vi "3_3_(2).vi"() -> ()   [LabVIEW 2012]
uses:
  Control 1.ctl
panel:
  in  "Таблиця 1 - Вхідні дані":string[][](table)
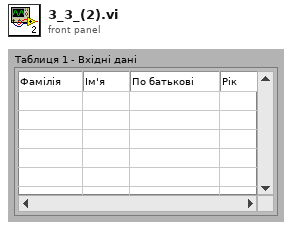
[diagram p1: front panel]
types:
  T1 = typedef "Control 1.ctl" = enum16{"Серверу", "Клієнту", "Зчитати", "Стоп", "1", "2", "3", "4"}
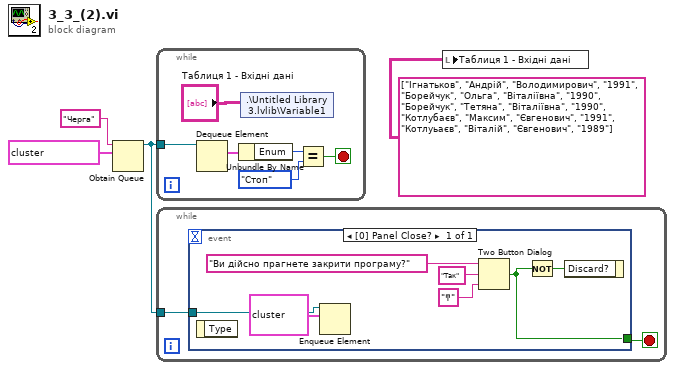
[diagram p0: block diagram]
diagram:
  n1 = Obtain Queue(name (unnamed)="Черга", element data type=cluster{"variant":variant, "Enum":T1} {"variant"=variant, "Enum"=enum."Стоп"}) -> (queue out=w2:refnum<queue>)  [unwired: 3 in, 2 out]
  n2 = while {
    tunnel: w2 -> [w10]
    stop <- w7 stop-if-true
    n3 = Dequeue Element(queue=w10) -> (element=w9:cluster{"variant":variant, "Enum":T1})  [unwired: 2 in, 3 out]
    n4 = Unbundle By Name(w9) -> ("Enum"=w6:T1)
    n5 = shared-variable ".\\Untitled Library 3.lvlib\\Variable1"("Таблиця 1 - Вхідні дані") -> ()  [unwired: 1 in, 1 out]
    n6 = Equal?(x=w6, y=Control_1."Стоп" ("Enum")) -> (x = y?=w7:bool)
  }
  n7 = while {
    tunnel: w2 -> [w11]
    stop <- w12 stop-if-true
    n8 = event shown="[0] Panel Close?" {
      selector: _ -> [_]
      dyn-events: _ -> [_]
      timeout: _ -> [_]
      tunnel: [w15] -> w12
      tunnel: w11 -> [w14]
      event Panel Close? {
        n9 = event-data() -> ()  [unwired: 1 in, 1 out]
        n10 = Enqueue Element(queue=w14, element=cluster{"variant":variant, "Enum":T1} {"variant"=variant, "Enum"=enum."Стоп"}) -> ()  [unwired: 2 in, 3 out]
        n11 = Two Button Dialog(message="Ви дійсно прагнете закрити програму?", 1:"ͳ" ("F button name (\"Cancel\")"), 2:"Так" ("T button name (\"OK\")")) -> (T button?=w15:bool)
        n12 = Not(x=w15) -> (.not. x?=w16:bool)
        n13 = event-data("Discard?"=w16) -> ()  [unwired: 1 in, 1 out]
      }
    }
  }
  n14 = local write "Таблиця 1 - Вхідні дані"(string[][] [["Ігнатьков", "Андрій", "Володимирович", "1991"], ["Борейчук", "Ольга", "Віталіївна", "1990"], ["Борейчук", "Тетяна", "Віталіївна", "1990"], ["Котлубаєв", "Максим", "Євгенович", "1991"], ["Котлуьаєв", "Віталій", "Євгенович", "1989"]] ("Таблиця 1")) -> ()
